vi "init.vi"(0 "Port Name":refnum<visa-resource-name>, 5 "COM response delay":u32, 7 "current error status":bool, 11 "error in":errorcluster) -> (1 "disk spinning disable state":T1(ring), 2 "new error status":bool, 3 "Disk position":bool, 4 "VISA resource name out":refnum<visa-resource-name>, 6 "Excitation Filter":u16(ring) items=["Unknown Filter 1", "Unknown Filter 2", "Unknown Filter 3", "Unknown Filter 4", "Unknown Filter 5", "Unknown Filter 6", "Unknown Filter 7", "Unknown Filter 8"], 8 "Emission Filter":u16(ring) items=["Unknown Filter 1", "Unknown Filter 2", "Unknown Filter 3", "Unknown Filter 4", "Unknown Filter 5", "Unknown Filter 6", "Unknown Filter 7", "Unknown Filter 8"], 9 "query response":string, 10 "Dichroic Mirror":u16(ring) items=["Unknown Filter 1", "Unknown Filter 2", "Unknown Filter 3", "Unknown Filter 4", "Unknown Filter 5"], 12 "Firmware Version":string, 13 "Shutter":bool, 14 "Disk spinning":bool, 15 "error out":errorcluster)   [LabVIEW 2016]
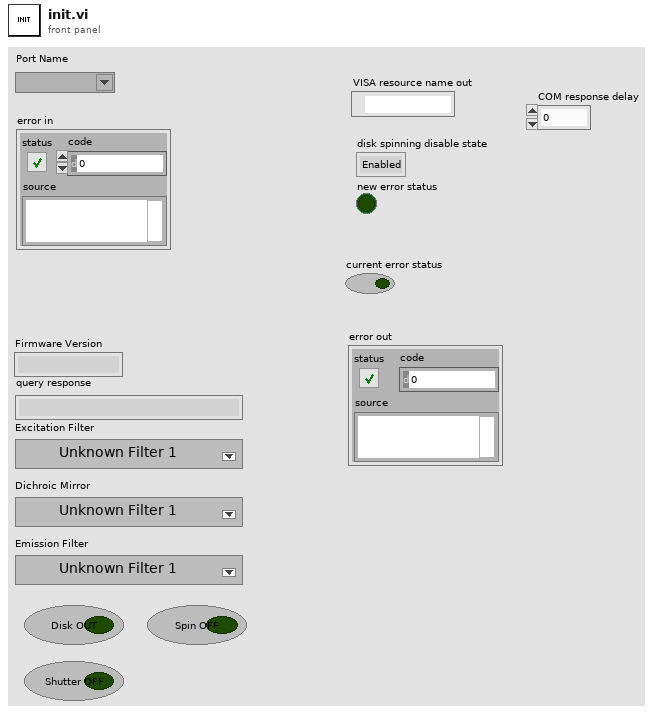
[diagram p1: front panel]
types:
  T1 = enum8{"Enabled", "Disabled", "Disabled and Grayed Out"}
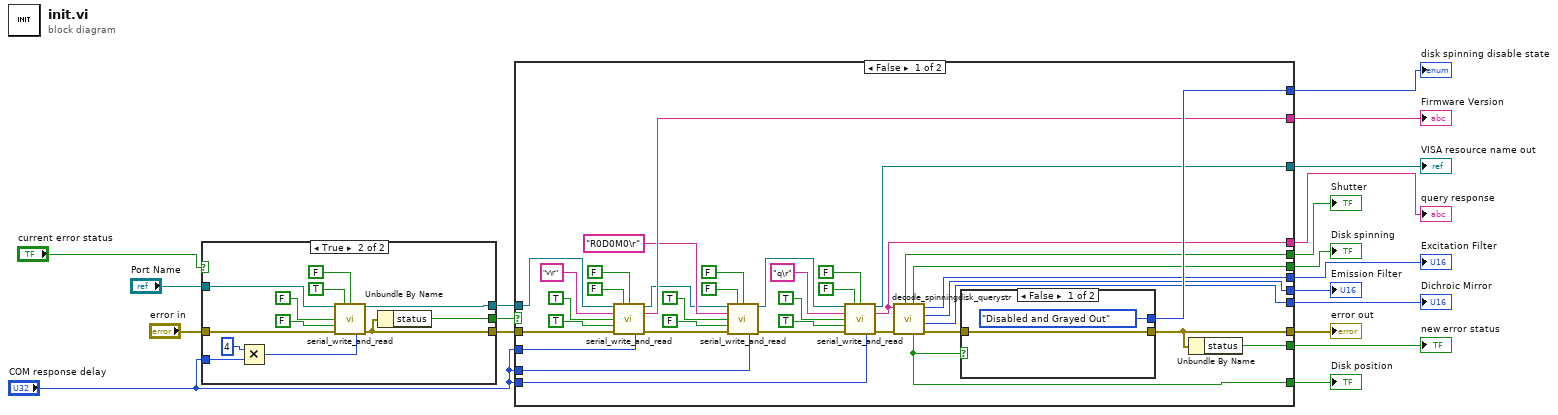
[diagram p0: block diagram]
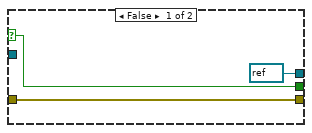
[diagram p2: hidden frame]
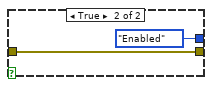
[diagram p3: hidden frame]
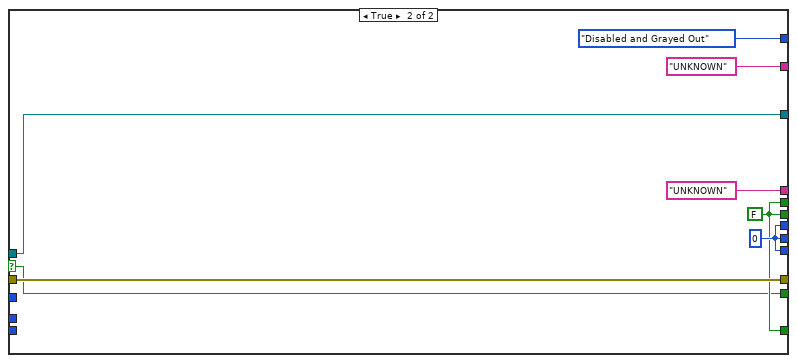
[diagram p4: hidden frame]
diagram:
  n1 = case shown="True" "current error status" {
    selector: "current error status" -> [w21 _]
    tunnel: [w22 w31] -> w17
    tunnel: "error in" -> [w22 w32]
    tunnel: [refnum<visa-resource-name> refnum ("VISA resource name out") w30] -> w18
    tunnel: [w21 w34] -> w19
    tunnel: "Port Name" -> [_ w33]
    tunnel: "COM response delay" -> [_ w25]
    frame False {
    }
    frame True {
      n2 = Multiply(x=u32 4, y=w25) -> (x*y=w24:u32)
      n3 = call "serial_write_and_read.vi"("port name in"=w33, "reconnect?"=TRUE, "disconnect?"=FALSE, "do writing?"=FALSE, "expecting response?"=FALSE, "error in"=w32, "COM response delay"=w24) -> ("port name out"=w30:refnum<visa-resource-name>, "error out"=w31:errorcluster)  [unwired: 6 in, 1 out]
      n4 = Unbundle By Name(w31) -> ("status"=w34:bool)
    }
  }
  n5 = case shown="False" w19 {
    selector: w19 -> [_ w79]
    tunnel: [w49 w84] -> w5
    tunnel: [w64 w83] -> w6
    tunnel: w18 -> [w60 w84]
    tunnel: w17 -> [w62 w83]
    tunnel: [w71 T1."Disabled and Grayed Out" ("Disabled")] -> w14
    tunnel: [w70 w80] -> w13
    tunnel: [w69 w80] -> w12
    tunnel: [w68 w82] -> w11
    tunnel: [w67 w82] -> w10
    tunnel: [w66 w82] -> w9
    tunnel: [w65 w80] -> w8
    tunnel: [w63 w79] -> w7
    tunnel: [w55 "UNKNOWN" ("read buffer")] -> w4
    tunnel: [w48 "UNKNOWN" ("read buffer")] -> w3
    tunnel: "COM response delay" -> [w37 _]
    tunnel: "COM response delay" -> [w36 _]
    tunnel: "COM response delay" -> [w35 _]
    frame False {
      n6 = call "serial_write_and_read.vi"("port name in"=w60, "reconnect?"=FALSE, "disconnect?"=FALSE, "write buffer"="v\r", "do writing?"=TRUE, "expecting response?"=TRUE, "error in"=w62, "COM response delay"=w37) -> ("port name out"=w41:refnum<visa-resource-name>, "read buffer"=w55:string, "error out"=w39:errorcluster)  [unwired: 5 in]
      n7 = call "serial_write_and_read.vi"("port name in"=w41, "reconnect?"=FALSE, "disconnect?"=FALSE, "write buffer"="R0D0M0\r", "do writing?"=TRUE, "expecting response?"=FALSE, "error in"=w39, "COM response delay"=w36) -> ("port name out"=w40:refnum<visa-resource-name>, "error out"=w38:errorcluster)  [unwired: 5 in, 1 out]
      n8 = call "serial_write_and_read.vi"("port name in"=w40, "reconnect?"=FALSE, "disconnect?"=FALSE, "write buffer"="q\r", "do writing?"=TRUE, "expecting response?"=TRUE, "error in"=w38, "COM response delay"=w35) -> ("port name out"=w49:refnum<visa-resource-name>, "read buffer"=w48:string, "error out"=w47:errorcluster)  [unwired: 5 in]
      n9 = call "decode_spinningdisk_querystr.vi"("input string"=w48, "error in"=w47) -> ("shutter"=w70:bool, "disk spinning"=w69:bool, "disk position"=w65:bool, "excitation filter"=w68:u16, "emission filter"=w67:u16, "dichroic mirror"=w66:u16, "error out"=w72:errorcluster)  [unwired: 2 in]
      n10 = case shown="False" w65 {
        tunnel: w72 -> [w74 w76]
        tunnel: [w74 w76] -> w64
        tunnel: [T1."Disabled and Grayed Out" ("Disabled") T1."Enabled" ("Disabled")] -> w71
        frame False {
        }
        frame True {
        }
      }
      n11 = Unbundle By Name(w64) -> ("status"=w63:bool)
    }
    frame True {
      w82 = u16 0 ("excitation filter")
      w80 = FALSE ("disk spinning")
    }
  }
  "disk spinning disable state" <- w14
  "Shutter" <- w13
  "Disk spinning" <- w12
  "Excitation Filter" <- w11
  "Emission Filter" <- w10
  "Dichroic Mirror" <- w9
  "Disk position" <- w8
  "new error status" <- w7
  "error out" <- w6
  "VISA resource name out" <- w5
  "Firmware Version" <- w4
  "query response" <- w3
